vi "CRYUpdate State by User Level.vi"   [LabVIEW 2013]
uses:
  CRYProject Editor Global.vi
  CRYCurveLibrary/Global/CRYCurve Library Global.vi
  CRYMainGlobal.vi
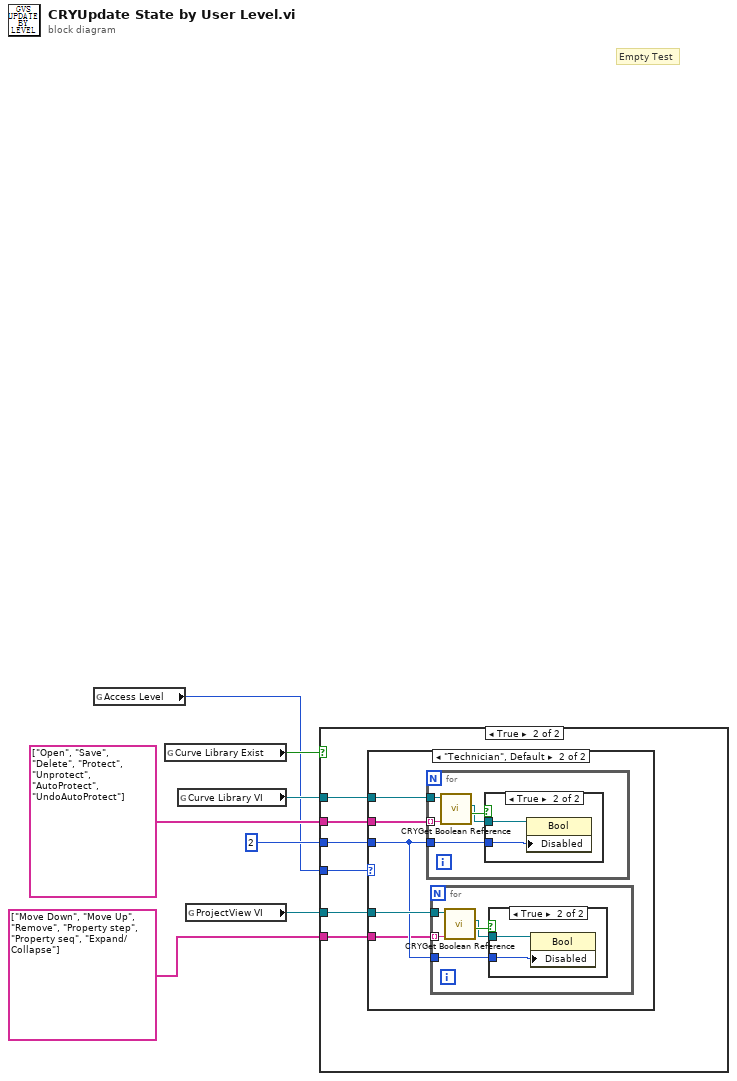
[diagram p0: block diagram]
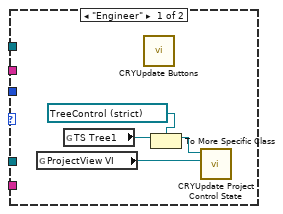
[diagram p3: hidden frame]
diagram:
  # "Empty Test"
  n1 = global read "CRYMainGlobal.vi" "Access Level"() -> (w1:enum16{"Engineer", "Technician", "Operator"})
  n2 = global read "CRYCurve Library Global.vi" "Curve Library Exist"() -> (w7:bool)
  n3 = global read "CRYCurve Library Global.vi" "Curve Library VI"() -> (w5:refnum<vi>)
  n4 = global read "CRYProject Editor Global.vi" "ProjectView VI"() -> (w4:refnum<vi>)
  n5 = case shown="True" w7 {
    tunnel: string[] ["Open", "Save", "Delete", "Protect", "Unprotect", "AutoProtect", "UndoAutoProtect"] ("Array") -> [_ w13]
    tunnel: w5 -> [_ w12]
    tunnel: u8 2 ("Disabled") -> [_ w10]
    tunnel: w4 -> [_ w11]
    tunnel: string[] ["Move Down", "Move Up", "Remove", "Property step", "Property seq", "Expand/Collapse"] ("Array") -> [_ w9]
    tunnel: w1 -> [_ w8]
    frame False {
    }
    frame True {
      n6 = case shown="\"Technician\", Default" w8 {
        tunnel: w13 -> [_ w22]
        tunnel: w12 -> [_ w21]
        tunnel: w11 -> [_ w20]
        tunnel: w10 -> [_ w19]
        tunnel: w9 -> [_ w18]
        frame "Engineer" {
          n7 = global read "CRYProject Editor Global.vi" "ProjectView VI"() -> (w17:refnum<vi>)
          n8 = global read "CRYProject Editor Global.vi" "TS Tree1"() -> (w16:refnum<vi>)
          n9 = call "CRYUpdate Buttons.vi"() -> ()  [unwired: 1 in, 11 out]
          n10 = To More Specific Class(target class=refnum<vi> refnum ("RefTree In"), reference=w16) -> (specific class reference=w14:refnum<vi>)  [unwired: 1 in, 1 out]
          n11 = call "CRYUpdate Project Control State.vi"("VI Ref"=w17, "RefTree In"=w14) -> ()  [unwired: 8 in, 2 out]
        }
        frame "Technician", Default {
          n12 = for {
            tunnel: w21 -> [w32]
            tunnel: w22 -> [w31] mode=indexing
            tunnel: w19 -> [w30]
            n13 = call "CRYGet Boolean Reference.vi"("Label Name"=w31, "VI Refnum"=w32) -> ("Exist?"=w34:bool, "Boolean Ref"=w33:refnum<vi>)  [unwired: 8 out]
            n14 = case shown="True" w34 {
              tunnel: w33 -> [_ w36]
              tunnel: w30 -> [_ w35]
              frame False {
              }
              frame True {
                n15 = property class="Bool"(reference=w36, "Disabled"=w35) -> ()  [unwired: 1 in, 2 out]
              }
            }
          }
          n16 = for {
            tunnel: w20 -> [w25]
            tunnel: w18 -> [w24] mode=indexing
            tunnel: w19 -> [w23]
            n17 = call "CRYGet Boolean Reference.vi"("Label Name"=w24, "VI Refnum"=w25) -> ("Exist?"=w27:bool, "Boolean Ref"=w26:refnum<vi>)  [unwired: 8 out]
            n18 = case shown="True" w27 {
              tunnel: w26 -> [_ w29]
              tunnel: w23 -> [_ w28]
              frame False {
              }
              frame True {
                n19 = property class="Bool"(reference=w29, "Disabled"=w28) -> ()  [unwired: 1 in, 2 out]
              }
            }
          }
        }
      }
    }
  }
